vi "Unitary_test_Escape_Unescape.vi"() -> (0 "Test OK":bool=TRUE)   [LabVIEW 2015]
panel:
  out "recovered string":string="hola\nvamos a probar\nsi esto tiene efecto o no  \\ \ny con comillas y todo \"\nahora cosas más exóticas\n\\n \n\\t \n\\\\n\n\"\n\\\"\n\"\"\\\n\n/*Para estabilizar arriba*/\nk1=-2.0;\nk2=35.0;\nk3=-1.5;\nk4=3.0;\n/*solo controlo ariba*/\nu[0]=-k1*(beta-consigna)-k2*alpha-k3*dbeta-k4*dalpha;\n\n/*para el swing up*/\nfunction sign(x) { return x > 0 ? 1 : x < 0 ? -1 : 1; }\nmu=50;//swing up gain\numax=6;\nEr=30.0/1000;\n\nMp=0.024;\nLp=0.127;\nJp=3.226e-5;\ng=9.81;\n\nMr=0.1;\nLr=0.095;\nR=6.3;\nkt=0.036;\n/*calculo la energía*/\nalpha2=alpha+Math.PI;\nEk = 0.5*Jp*dalpha*dalpha;\nEp = 0.5*Mp*g*Lp*(1-Math.cos(alpha2));\nE = Ek+Ep;\n/*y ahora el control*/\ntau=sign(Math.cos(alpha2)*dalpha)*mu*(E-Er);\n/*saturo*/\n//if (tau<-umax) tau=-umax;\n//if (tau>umax) tau=umax;\n/*por fin calculo u*/\nus=Mr*Lr*R*tau/kt\n\n//uso uno u otro dependiendo del ángulo (20 grados)\nif (Math.abs(alpha)>0.35) {u[0]=us;}\n//saco la energia para verla\nu[1]=E;\n"
  in  "String":string="hola\nvamos a probar\nsi esto tiene efecto o no  \\ \ny con comillas y todo \"\nahora cosas más exóticas\n\\n \n\\t \n\\\\n\n\"\n\\\"\n\"\"\\\n\n/*Para estabilizar arriba*/\nk1=-2.0;\nk2=35.0;\nk3=-1.5;\nk4=3.0;\n/*solo controlo ariba*/\nu[0]=-k1*(beta-consigna)-k2*alpha-k3*dbeta-k4*dalpha;\n\n/*para el swing up*/\nfunction sign(x) { return x > 0 ? 1 : x < 0 ? -1 : 1; }\nmu=50;//swing up gain\numax=6;\nEr=30.0/1000;\n\nMp=0.024;\nLp=0.127;\nJp=3.226e-5;\ng=9.81;\n\nMr=0.1;\nLr=0.095;\nR=6.3;\nkt=0.036;\n/*calculo la energía*/\nalpha2=alpha+Math.PI;\nEk = 0.5*Jp*dalpha*dalpha;\nEp = 0.5*Mp*g*Lp*(1-Math.cos(alpha2));\nE = Ek+Ep;\n/*y ahora el control*/\ntau=sign(Math.cos(alpha2)*dalpha)*mu*(E-Er);\n/*saturo*/\n//if (tau<-umax) tau=-umax;\n//if (tau>umax) tau=umax;\n/*por fin calculo u*/\nus=Mr*Lr*R*tau/kt\n\n//uso uno u otro dependiendo del ángulo (20 grados)\nif (Math.abs(alpha)>0.35) {u[0]=us;}\n//saco la energia para verla\nu[1]=E;\n"
  out "x-y":u32
  out "Json_string":string="hola\\fvamos a probar\\fsi esto tiene efecto o no  \\\\ \\fy con comillas y todo \\\"\\fahora cosas más exóticas\\f\\\\n \\f\\\\t \\f\\\\\\\\n\\f\\\"\\f\\\\\\\"\\f\\\"\\\"\\\\\\f\\f/*Para estabilizar arriba*/\\fk1=-2.0;\\fk2=35.0;\\fk3=-1.5;\\fk4=3.0;\\f/*solo controlo ariba*/\\fu[0]=-k1*(beta-consigna)-k2*alpha-k3*dbeta-k4*dalpha;\\f\\f/*para el swing up*/\\ffunction sign(x) { return x > 0 ? 1 : x < 0 ? -1 : 1; }\\fmu=50;//swing up gain\\fumax=6;\\fEr=30.0/1000;\\f\\fMp=0.024;\\fLp=0.127;\\fJp=3.226e-5;\\fg=9.81;\\f\\fMr=0.1;\\fLr=0.095;\\fR=6.3;\\fkt=0.036;\\f/*calculo la energía*/\\falpha2=alpha+Math.PI;\\fEk = 0.5*Jp*dalpha*dalpha;\\fEp = 0.5*Mp*g*Lp*(1-Math.cos(alpha2));\\fE = Ek+Ep;\\f/*y ahora el control*/\\ftau=sign(Math.cos(alpha2)*dalpha)*mu*(E-Er);\\f/*saturo*/\\f//if (tau<-umax) tau=-umax;\\f//if (tau>umax) tau=umax;\\f/*por fin calculo u*/\\fus=Mr*Lr*R*tau/kt\\f\\f//uso uno u otro dependiendo del ángulo (20 grados)\\fif (Math.abs(alpha)>0.35) {u[0]=us;}\\f//saco la energia para verla\\fu[1]=E;\\f"
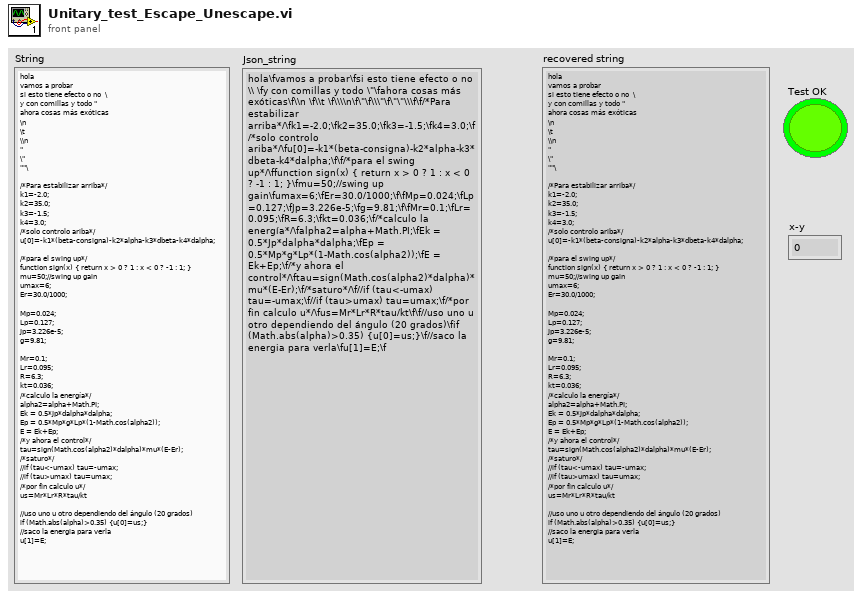
[diagram p1: front panel]
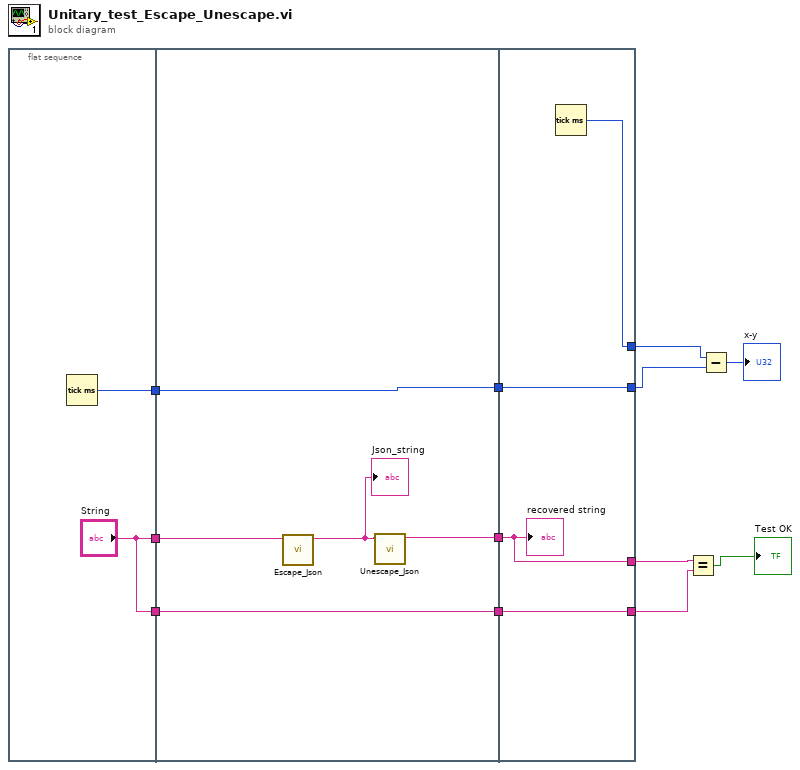
[diagram p0: block diagram]
diagram:
  n1 = flat-sequence {
    tunnel: [w14] -> w11
    tunnel: ["String"] -> w7
    tunnel: ["String"] -> w4
    tunnel: [w19] -> w12
    tunnel: w11 -> [w19]
    tunnel: w7 -> [w18]
    tunnel: [w16] -> w6
    tunnel: w4 -> [w15]
    tunnel: [w15] -> w3
    tunnel: [w23] -> w9
    tunnel: w12 -> [w23]
    tunnel: [w22] -> w10
    tunnel: w6 -> [w21]
    tunnel: [w21] -> w5
    tunnel: w3 -> [w20]
    tunnel: [w20] -> w2
    frame #0 {
      n2 = Tick Count (ms)() -> (millisecond timer value=w14:u32)
    }
    frame #1 {
      n3 = call "Escape_Json.vi"("String"=w18) -> ("Json_string"=w17:string)  [unwired: 9 in]
      "Json_string" <- w17
      n4 = call "Unescape_Json.vi"("Json_String"=w17) -> ("String"=w16:string)  [unwired: 9 in]
    }
    frame #2 {
      n5 = Tick Count (ms)() -> (millisecond timer value=w22:u32)
      "recovered string" <- w21
    }
  }
  n6 = Equal?(x=w5, y=w2) -> (x = y?=→"Test OK":bool)
  n7 = Subtract(x=w10, y=w9) -> (x-y=→"x-y":u32)
